vi "SURFTdll.vi"(8 "error in (no error)":errorcluster, 11 "Inputs":cluster{"t":dbl, "D":dbl, "z":dbl[]}) -> (0 "error out":errorcluster, 3 "Outputs":T1)   [LabVIEW 2015]
doc: "subroutine SURFTdll(t, D, z, sigma, ierr, herr, herr_length)\n\nTwo similar routines are provided for calculating surface tension.\nSURTEN is more efficient if the liquid and vapor density and composition\nare known (e.g., from a previous call to SATT). If these are not known,\nthen SURFT may be used.\n\nINPUTS:\nt -- Temperature [K]\nD -- molar density of liquid phase [mol/L]. If D > 0 use D as an input value. D < 0 call SATT to find density\nz -- composition of liquid phase [array of mol frac]\n\nOUTPUTS:\nD -- molar density of liquid phase [mol/L]. If D > 0 use D as an input value. D < 0 call SATT to find density.\nsigma --Surface tension [N/m]\nierr -- Error flag: 0 - Successful other error messages returned from SATT or STN\n 1 = T < Tmin\n 8 = x out of range\n 9 = T and x out of range\n 120 = CRITP did not converge\n 121 = T > Tcrit\n 122 = TPRHO-liquid did not converge in SATT\n 123 = TPRHO-vapor did not converge in SATT\n 124 = SATT pure fluid iteration did not converge\n 128 = SATT mixture iteration did not converge\nherr -- Error string (character*255)\nherr_length -- length of variable herr (default: 255)"
uses:
  REFPROP.dll
panel:
  # "REFPROP-SURFTdll.vi"
  # "void  SURFTdll(double *t, double *D, double *z, double *sigma, int32_t *ierr, CStr herr, int32_t herr_length)"
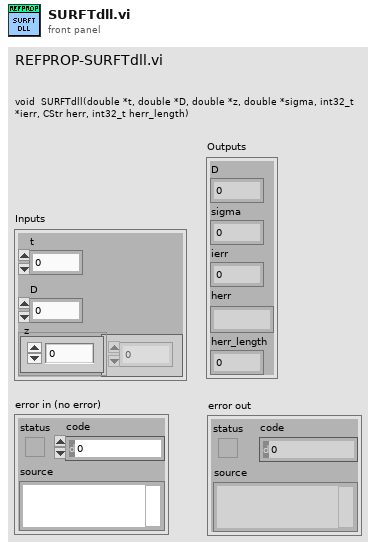
[diagram p1: front panel]
types:
  T1 = cluster{"D":dbl, "sigma":dbl, "ierr":i32, "herr":string, "herr_length":i32}
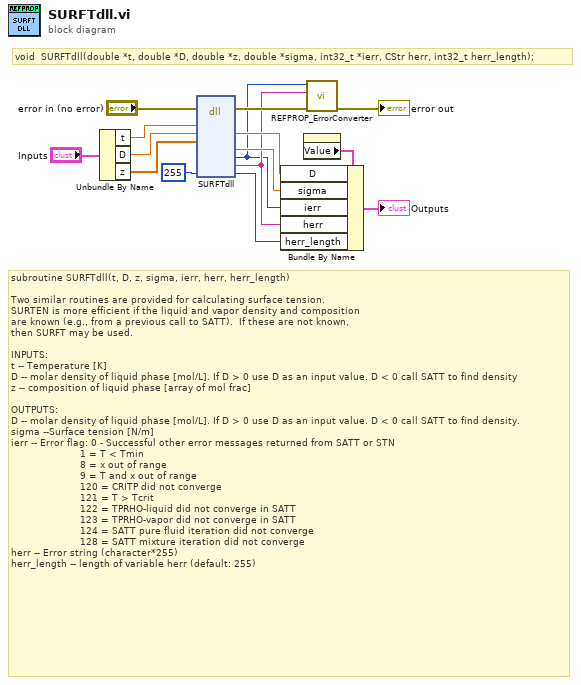
[diagram p0: block diagram]
diagram:
  # "void  SURFTdll(double *t, double *D, double *z, double *sigma, int32_t *ierr, CStr herr, int32_t herr_length);"
  # "subroutine SURFTdll(t, D, z, sigma, ierr, herr, herr_length)\n\nTwo similar routines are provided for calculating surface tension.\nSURTEN is more efficient if the liquid and vapor density and composition\nare known (e.g., from a previous call to SATT).  If these are not known,\nthen SURFT may be used.\n\nINPUTS:\nt -- Temperature [K]\nD -- molar density of liquid phase [mol/L]. If D > 0 use D as an input value. D < 0 call SATT to find density\nz -- composition of liquid phase [array of mol frac]\n\nOUTPUTS:\nD -- molar density of liquid phase [mol/L]. If D > 0 use D as an input value. D < 0 call SATT to find density.\nsigma --Surface tension [N/m]\nierr -- Error flag: 0 - Successful other error messages returned from SATT or STN\n                       1 = T < Tmin\n                       8 = x out of range\n                       9 = T and x out of range\n                       120 = CRITP did not converge\n                       121 = T > Tcrit\n                       122 = TPRHO-liquid did not converge in SATT\n                       123 = TPRHO-vapor did not converge in SATT\n                       124 = SATT pure fluid iteration did not converge\n                       128 = SATT mixture iteration did not converge\nherr -- Error string (character*255)\nherr_length -- length of variable herr (default: 255)"
  n1 = Unbundle By Name("Inputs") -> ("t"=w9:dbl, "D"=w10:dbl, "z"=w11:dbl[])
  n2 = dll-call lib="C:/Users/lauria/Desktop/REFPROP 10 LabVIEW Wrapper BETA/REFPROP/REFPROP.*" fn="SURFTdll"(error in="error in (no error)", "t"=w9, "D"=w10, "z"=w11, "herr_length"=255 ("ln")) -> (error out=w14:errorcluster, "D"=w5:dbl, "sigma"=w4:dbl, "ierr"=w1:i32, "herr"=w2:string, "herr_length"=w3:i32)  [unwired: 8 in, 1 out]
  n3 = property on="Outputs" class="Clust (strict)"() -> ("Value"=w6:T1)  [unwired: 2 in, 2 out]
  n4 = Bundle By Name(cluster=w6, "D"=w5, "sigma"=w4, "ierr"=w1, "herr"=w2, "herr_length"=w3) -> (→"Outputs":T1)
  n5 = call "REFPROP_ErrorConverter.vi"("error in (no error)"=w14, "Error Message"=w2, "Error Code"=w1) -> ("error out"=→"error out":errorcluster)  [unwired: 8 in]
